vi "Actor Core.vi"(8 "error in":errorcluster, 11 "Synchronization Device in":refnum<class "Synchronization Device.lvclass">) -> (0 "error out":errorcluster, 3 "Actor out":refnum<class "Actor.lvclass">)   [LabVIEW 2018, in "Synchronization Device.lvlib" / "Synchronization Device.lvclass"]
doc: "(<B>Filename</B>: Actor Framework.lvlib:Actor.lvclass:Actor Core.vi)\n\nReceives messages to the actor, reacts to them, and initiates any error handling that may shut the actor down.\n\nDescendant classes may override this VI to append parallel tasks for the actor to complete while it handles messages. Overrides use the Call Parent Method node."
uses:
  Synchronization Device.lvclass
  <vilib>/ActorFramework/Actor/Actor.lvclass
  Synchronization Device.lvclass/Synchronization Device.ctl
  <vilib>/DAQmx/write.llb/DAQmx Write (Digital 1D Bool 1Chan 1Samp).vi
  <vilib>/DAQmx/miscellaneous.llb/DAQmx Fill In Error Info.vi
  Device/Device.lvclass
panel:
  in  "Stop Button":bool
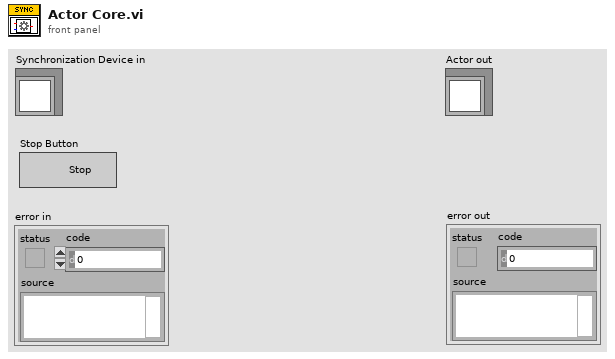
[diagram p1: front panel]
types:
  T1 = cluster{"Interval (ms)":dbl, "ALEX":bool, "Shutter Enable":bool[], "Stream":bool, "Duty Cycle":dbl}
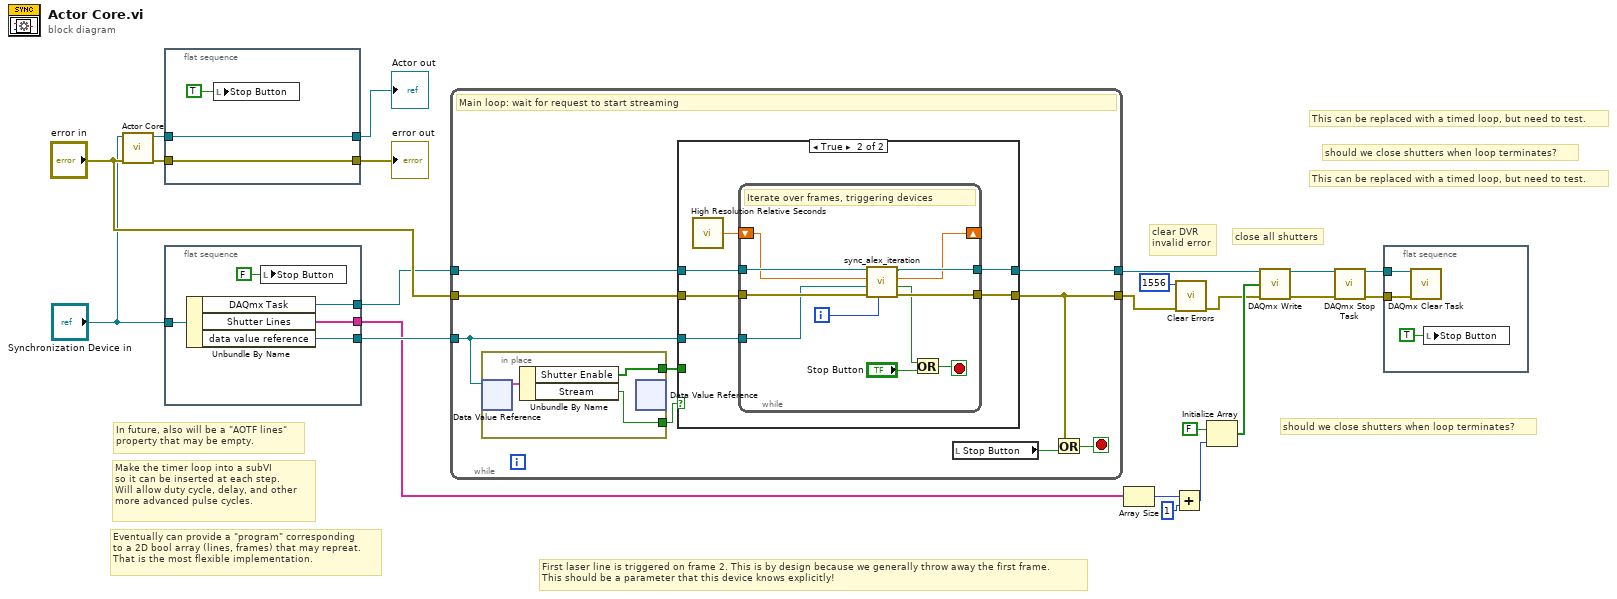
[diagram p0: block diagram]
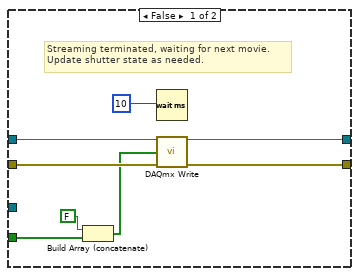
[diagram p2: hidden frame]
diagram:
  # "First laser line is triggered on frame 2. This is by design because we generally throw away the first frame.\nThis should be a parameter that this device knows explicitly!"
  # "should we close shutters when loop terminates?"
  # "This can be replaced with a timed loop, but need to test."
  # "This can be replaced with a timed loop, but need to test."
  # "should we close shutters when loop terminates?"
  # "Eventually can provide a \"program\" corresponding\nto a 2D bool array (lines, frames) that may repreat.\nThat is the most flexible implementation."
  # "Make the timer loop into a subVI\nso it can be inserted at each step.\nWill allow duty cycle, delay, and other\nmore advanced pulse cycles."
  # "In future, also will be a \"AOTF lines\"\nproperty that may be empty."
  # "close all shutters"
  # "clear DVR\ninvalid error"
  n1 = call-parent "Actor Core.vi"("error in"="error in", "Device in"="Synchronization Device in") -> ("error out"=w19:errorcluster, "Actor out"=w22:refnum<class "Actor.lvclass">)  [unwired: 8 in]
  n2 = flat-sequence {
    tunnel: w22 -> [w25]
    tunnel: [w25] -> w21
    tunnel: [w24] -> w20
    tunnel: w19 -> [w24]
    frame #0 {
      n3 = local write "Stop Button"(TRUE) -> ()
    }
  }
  n4 = flat-sequence {
    tunnel: "Synchronization Device in" -> [w30]
    tunnel: [w29] -> w12
    tunnel: [w28] -> w9
    tunnel: [w27] -> w13
    frame #0 {
      n5 = Unbundle By Name(w30) -> ("DAQmx Task"=w28:refnum<k21>, "Shutter Lines"=w29:string[], "data value reference"=w27:refnum<data-value>)
      n6 = local write "Stop Button"(FALSE ("Stop Button")) -> ()
    }
  }
  n7 = while {
    tunnel: w13 -> [w33]
    tunnel: w9 -> [w37]
    tunnel: [w38] -> w17
    tunnel: "error in" -> [w39]
    tunnel: [w35] -> w16
    stop <- w36 stop-if-true
    # "Main loop: wait for request to start streaming"
    n8 = in-place {
      in-place-border: [w41] -> w34
      in-place-border: [w40] -> w32
      n9 = in-place-dvr #1(w33) -> (w42:T1)  [unwired: 1 out]
      n10 = Unbundle By Name(w42) -> ("Shutter Enable"=w40:bool[], "Stream"=w41:bool)
      n11 = in-place-dvr #1() -> ()  [unwired: 1 in, 2 out]
    }
    n12 = case shown="True" w34 {
      tunnel: w39 -> [w47 w52]
      tunnel: [w49 w55] -> w38
      tunnel: w33 -> [_ w51]
      tunnel: w37 -> [w46 w53]
      tunnel: [w48 w54] -> w35
      tunnel: w32 -> [w44 _]
      frame False {
        # "Streaming terminated, waiting for next movie.\nUpdate shutter state as needed."
        n13 = Build Array (concatenate)(FALSE, w44) -> (w45:bool[])
        n14 = Wait (ms)(milliseconds to wait=u32 10 ("millisecond multiple")) -> ()  [unwired: 1 out]
        n15 = call-poly <vilib>:"DAQmx Write.vi"("task/channels in"=w46, "data"=w45, "error in"=w47) -> ("task out"=w49:refnum<k21>, "error out"=w48:errorcluster)  [unwired: 10 in, 1 out]
      }
      frame True {
        n16 = call <vilib>:"High Resolution Relative Seconds.vi"() -> ("relative seconds"=w56:dbl)
        n17 = while {
          tunnel: w53 -> [w64]
          tunnel: [w66] -> w55
          shift-right: [w65] -> _
          shift-left: w56 -> [w62]
          tunnel: [w67] -> w54
          tunnel: w52 -> [w63]
          tunnel: w51 -> [w58]
          i -> [w57]
          stop <- w61 stop-if-true
          # "Iterate over frames, triggering devices"
          n18 = call "sync_alex_iteration.vi"("frame number"=w57, "error in"=w63, "data value reference"=w58, "last frame (s)"=w62, "DAQmx Task"=w64) -> ("error out"=w67:errorcluster, "Stop?"=w59:bool, "relative seconds 2"=w65:dbl, "task out"=w66:refnum<k21>)  [unwired: 1 in]
          n19 = Or(x=w59, y="Stop Button") -> (x .or. y?=w61:bool)
        }
      }
    }
    n20 = local read "Stop Button"() -> (w31:bool)
    n21 = Or(x=w35, y=w31) -> (x .or. y?=w36:bool)
  }
  n22 = Array Size(array=w12) -> (size(s)=w14:i32)
  n23 = Add(x=w14, y=1) -> (x+y=w5:i32)
  n24 = call <vilib>:"Clear Errors.vi"("error in (no error)"=w16, "specific error code to clear (0: all)"=1556) -> ("error out"=w4:errorcluster)  [unwired: 4 in, 1 out]
  n25 = Initialize Array(FALSE ("element"), w5) -> (w7:bool[])
  n26 = call-poly <vilib>:"DAQmx Write.vi"("task/channels in"=w17, "data"=w7, "error in"=w4) -> ("task out"=w11:refnum<k21>, "error out"=w10:errorcluster)  [unwired: 10 in, 1 out]
  n27 = call <vilib>:"DAQmx Stop Task.vi"("task/channels in"=w11, "error in"=w10) -> ("task out"=w2:refnum<k21>, "error out"=w1:errorcluster)  [unwired: 12 in]
  n28 = flat-sequence {
    tunnel: w2 -> [w70]
    tunnel: w1 -> [w69]
    frame #0 {
      n29 = call <vilib>:"DAQmx Clear Task.vi"("task in"=w70, "error in"=w69) -> ()  [unwired: 13 in, 1 out]
      n30 = local write "Stop Button"(TRUE ("Stop Button")) -> ()
    }
  }
  "error out" <- w20
  "Actor out" <- w21
